vi "Write Stdin.vi"(8 "error in":errorcluster, 10 "write buffer":string, 11 "pipe in":T1) -> (0 "error out":errorcluster, 2 "return count":i32, 3 "pipe out":T1)   [LabVIEW 2020, in "LV Process library.lvlib"]
doc: "Calls lv_proc.dll to write string buffer to stdin of a process and returns written count.\n\n---\nLV Process works only with lv_proc.dll library, which is part of vipm package or should be delivered together with packed library. Placement of this dll is selected in terminal of Create Process.vi."
uses:
  LV Process library.lvlib
  Pipe Handle.ctl
  <vilib>/Utility/error.llb/Error Cluster From Error Code.vi
  <vilib>/ErrorRing/Error Ring.xnode
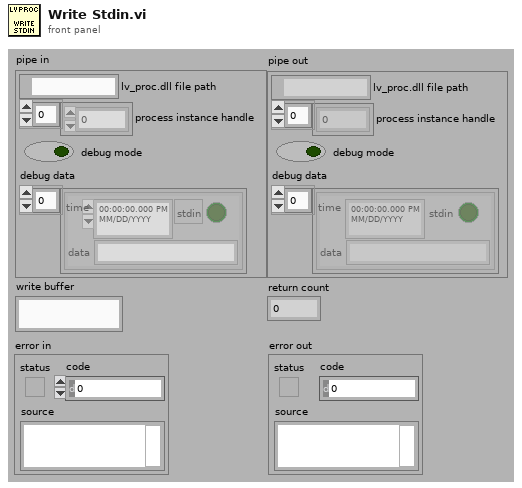
[diagram p1: front panel]
types:
  T1 = typedef "LV Process library.lvlib/Pipe Handle.ctl" = cluster{"lv_proc.dll file path":path, "process instance handle":u32[], "debug mode":bool, "debug data":cluster{"time":timestamp, "stdin":bool, "data":string}[]}
  T2 = cluster{"time":timestamp, "stdin":bool, "data":string}[]
  T3 = cluster{"time":timestamp, "stdin":bool, "data":string}
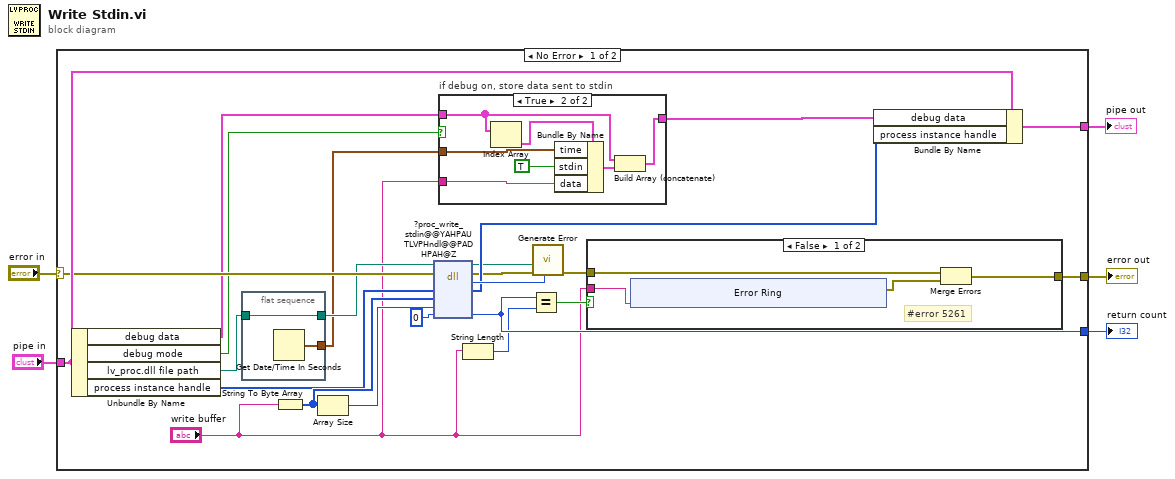
[diagram p0: block diagram]
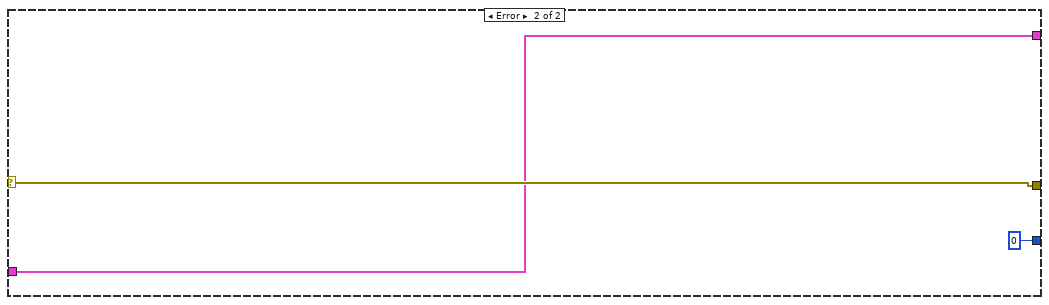
[diagram p4: hidden frame]
diagram:
  n1 = case shown="No Error" "error in" {
    selector: "error in" -> [w18 w53]
    tunnel: [w17 0 ("written")] -> w5
    tunnel: [w24 w51] -> w4
    tunnel: "pipe in" -> [w23 w51]
    tunnel: [w13 w53] -> w2
    frame No Error {
      n2 = Unbundle By Name(w23) -> ("debug data"=w11:T2, "debug mode"=w12:bool, "lv_proc.dll file path"=w9:path, "process instance handle"=w21:u32[])
      n3 = flat-sequence {
        tunnel: [w30] -> w10
        tunnel: w9 -> [w30]
        tunnel: [w29] -> w8
        frame #0 {
          n4 = Get Date/Time In Seconds() -> (seconds since 1Jan1904=w29:timestamp)
        }
      }
      n5 = String To Byte Array(string="write buffer") -> (unsigned byte array=w27:u8[])
      n6 = Array Size(array=w27) -> (size(s)=w26:i32)
      n7 = dll-call lib="C:/Data/GOLPI/LV Process/lv_proc.dll" fn="?proc_write_stdin@@YAHPAUTLVPHndl@@PADHPAH@Z" label="proc_write_stdin"(path in=w10, error in=w18, "proc"=w21, "buffer"=w27, "size"=w26, "written"=0 ("written mem")) -> (path out=w20:path, error out=w19:errorcluster, "error"=w25:i32, "proc"=w22:u32[], "written"=w17:i32)  [unwired: 3 in]
      n8 = case "if debug on, store data sent to stdin" shown="True" w12 {
        tunnel: w11 -> [w31 w37]
        tunnel: w8 -> [_ w34]
        tunnel: "write buffer" -> [_ w33]
        tunnel: [w31 w32] -> w6
        frame False {
        }
        frame True {
          n9 = Index Array(array=w37) -> (element=w38:T3)  [unwired: 1 in]
          n10 = Bundle By Name(cluster=w38, "time"=w34, "stdin"=TRUE, "data"=w33) -> (w36:T3)
          n11 = Build Array (concatenate)(w37, w36) -> (w32:T2)
        }
      }
      n12 = String Length(string="write buffer") -> (length=w16:i32)
      n13 = Equal?(x=w17, y=w16) -> (x = y?=w15:bool)
      n14 = call "Generate Error.vi"("error code in"=w25, "error in"=w19, "lv_proc.dll path in"=w20) -> ("error out"=w14:errorcluster)  [unwired: 6 in, 1 out]
      n15 = case shown="False" w15 {
        tunnel: w14 -> [w42 w50]
        tunnel: [w40 w50] -> w13
        tunnel: "write buffer" -> [w39 _]
        frame False {
          # "#error 5261"
          n16 = xnode "Error Ring"("parameter 0"=w39) -> ("error out"=w41:errorcluster)
          n17 = Merge Errors(w42, w41) -> (w40:errorcluster)
        }
        frame True {
        }
      }
      n18 = Bundle By Name(cluster=w23, "debug data"=w6, "process instance handle"=w22) -> (w24:T1)
    }
    frame Error {
    }
  }
  "error out" <- w2
  "return count" <- w5
  "pipe out" <- w4
